vi "readFromXML.vi"(8 "error in (no error)":errorcluster, 10 "XML in":string, 11 "IAA in":refnum<class "IAA.lvclass">) -> (0 "error out":errorcluster, 3 "IAA out":refnum<class "IAA.lvclass">)   [LabVIEW 2009, in "IAA.lvclass"]
uses:
  IAA.lvclass
  Common/UnitsAndXML/FlattenItemWithUnitToXML/FlattenPlaneAngleToXML/PlaneAngleUnit.ctl
  IAA.lvclass/IAA.ctl
  Common/UnitsAndXML/UnflattenItemWithUnitFromXML/UnflattenPlaneAngleFromXML/typeMethods/unflattenPlaneAngleFromXML_Scalar.vi
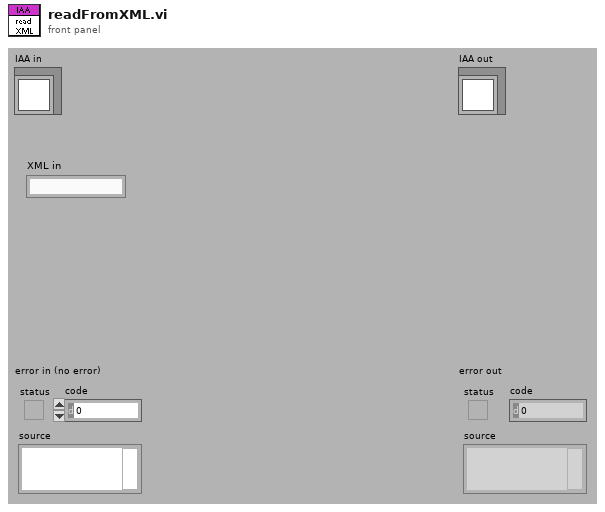
[diagram p1: front panel]
types:
  T1 = typedef "PlaneAngleUnit.ctl" = enum16{"rad", "deg", "'", "\""}
  T2 = typedef "XML element.ctl" = cluster{"name":string, "contents":string}
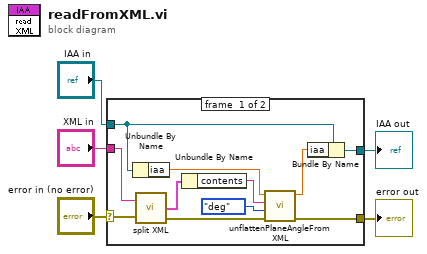
[diagram p0: block diagram]
diagram:
  n1 = case shown="No Error" "error in (no error)" {
    selector: "error in (no error)" -> [w15 w18]
    tunnel: [w7 w18] -> w4
    tunnel: [w12 w17] -> w2
    tunnel: "IAA in" -> [w13 w17]
    tunnel: "XML in" -> [w16 _]
    frame #0 {
      n2 = Unbundle By Name(w13) -> ("iaa"=w11:dbl[unit])
      n3 = call "split XML.vi"("XMLString in"=w16, "error in (no error)"=w15) -> ("XML element"=w14:T2, "error out"=w8:errorcluster)  [unwired: 1 out]
      n4 = Unbundle By Name(w14) -> ("contents"=w10:string)
      n5 = call-poly "unflattenPlaneAngleFromXML.vi"("error in (no error)"=w8, "planeAngleUnitInXML"=PlaneAngleUnit."deg", "xmlString"=w10, "planeAngleForType"=w11) -> ("error out"=w7:errorcluster, "planeAngle"=w6:dbl[unit])  [unwired: 6 in]
      n6 = Bundle By Name(cluster=w13, "iaa"=w6) -> (w12:refnum<class "IAA.lvclass">)
    }
    frame #1 {
    }
  }
  "error out" <- w4
  "IAA out" <- w2
